vi "Gradient.vi"(7 "Percent":dbl=1.0, 10 "End Color":u32(colorbox)=16777238, 11 "Start Color":u32(colorbox)) -> (3 "Gradient Color":u32(colorbox))   [LabVIEW 2020, in "ColorSelector.lvclass"]
doc: "This VI uses the RGB values of two colors to represent points in a 3-D space and then calculates a line between the two points. The \"Percent\" (0-1) is the percent distance along this line from the Start Color to the End Color.\n<b> </b> <b> </b>\n©2017 Q Software Innovations, LLC (QSI)\nwritten by Quentin Alldredge\nproduced in LabVIEW 2015\n\nsupport@qsoftwareinnovations.com\nwww.qsoftwareinnovations.com\n\nAll rights reserved.\n\nRedistribution and use in source and binary forms, with or without modification, are permitted provided that the following conditions are met:\n\n * Redistributions of source code must retain the above copyright notice, this list of conditions and the following disclaimer.\n * Redistributions in binary form must reproduce the above copyright notice, this list of conditions and the following disclaimer in the documentation and/or other materials provided with the distribution.\n * Neither the name of Q Software Innovations, LLC. nor the names of its contributors may be used to endorse or promote products derived from this software without specific prior written permission.\n\nTHIS SOFTWARE IS PROVIDED BY THE COPYRIGHT HOLDERS AND CONTRIBUTORS \"AS IS\" AND ANY EXPRESS OR IMPLIED WARRANTIES, INCLUDING, BUT NOT LIMITED TO, THE IMPLIED WARRANTIES OF MERCHANTABILITY AND FITNESS FOR A PARTICULAR PURPOSE ARE DISCLAIMED. IN NO EVENT SHALL THE COPYRIGHT OWNER OR CONTRIBUTORS BE LIABLE FOR ANY DIRECT, INDIRECT, INCIDENTAL, SPECIAL, EXEMPLARY, OR CONSEQUENTIAL DAMAGES (INCLUDING, BUT NOT LIMITED TO, PROCUREMENT OF SUBSTITUTE GOODS OR SERVICES; LOSS OF USE, DATA, OR PROFITS; OR BUSINESS INTERRUPTION) HOWEVER CAUSED AND ON ANY THEORY OF LIABILITY, WHETHER IN CONTRACT, STRICT LIABILITY, OR TORT (INCLUDING NEGLIGENCE OR OTHERWISE) ARISING IN ANY WAY OUT OF THE USE OF THIS SOFTWARE, EVEN IF ADVISED OF THE POSSIBILITY OF SUCH DAMAGE."
uses:
  ColorSelector.lvclass
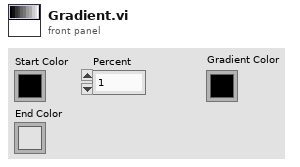
[diagram p1: front panel]
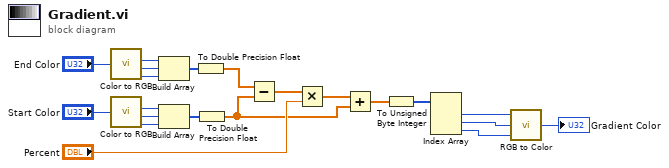
[diagram p0: block diagram]
diagram:
  n1 = call <vilib>:"Color to RGB.vi"("Color"="End Color") -> ("R"=w19:u8, "G"=w18:u8, "B"=w17:u8)  [unwired: 1 out]
  n2 = call <vilib>:"Color to RGB.vi"("Color"="Start Color") -> ("R"=w16:u8, "G"=w15:u8, "B"=w14:u8)  [unwired: 1 out]
  n3 = Build Array(w19, w18, w17) -> (w13:u8[])
  n4 = Build Array(w16, w15, w14) -> (w12:u8[])
  n5 = To Double Precision Float(number=w13) -> (double precision float=w10:dbl[])
  n6 = To Double Precision Float(number=w12) -> (double precision float=w5:dbl[])
  n7 = Subtract(x=w10, y=w5) -> (x-y=w6:dbl[])
  n8 = Multiply(x=w6, y="Percent") -> (x*y=w4:dbl[])
  n9 = Add(x=w4, y=w5) -> (x+y=w3:dbl[])
  n10 = To Unsigned Byte Integer(number=w3) -> (unsigned 8bit integer=w7:u8[])
  n11 = Index Array(array=w7) -> (element #1=w9:u8, element #2=w2:u8, element #3=w1:u8)  [unwired: 3 in]
  n12 = call <vilib>:"RGB to Color.vi"("B"=w1, "G"=w2, "R"=w9) -> ("Color"=→"Gradient Color":u32)
